vi "Set google_protobuf_Type.vi"(7 "Complete Call (T)":bool=TRUE, 8 "error in (no error)":errorcluster, 10 "package_templatemessage":T1, 11 "gRPCid":T9) -> (0 "error out":errorcluster)   [LabVIEW 2020, in "Measurement Plugin Measurement Server Internal.lvlib"]
uses:
  Measurement Plugin Measurement Server Internal.lvlib
  <vilib>/gRPC/LabVIEW gRPC Library/Shared/grpcId.ctl
  google_protobuf_Type.ctl
  google_protobuf_Field.ctl
  google_protobuf_Field_Kind.ctl
  google_protobuf_Field_Cardinality.ctl
  google_protobuf_Option.ctl
  google_protobuf_Any.ctl
  google_protobuf_SourceContext.ctl
  google_protobuf_Syntax.ctl
  google_protobuf_Type_Flat.ctl
  google_protobuf_Field_Flat.ctl
  google_protobuf_Option_Flat.ctl
  google_protobuf_Any_Flat.ctl
  google_protobuf_SourceContext_Flat.ctl
  dcc74a39-081a-4bdd-860b-8ed792803c96.vi
  RichToFlatgoogle_protobuf_Field.vi
  RichToFlatgoogle_protobuf_Option.vi
  RichToFlatgoogle_protobuf_SourceContext.vi
  <vilib>/gRPC/LabVIEW gRPC Library/Shared/TranslateGrpcError.vi
  RichToFlatgoogle_protobuf_Any.vi
  <vilib>/gRPC/LabVIEW gRPC Library/Server API/Server/Get Server DLL Path.vi
  <vilib>/Utility/error.llb/Error Cluster From Error Code.vi
  <vilib>/Utility/error.llb/Simple Error Handler.vi
  <vilib>/gRPC/LabVIEW gRPC Library/grpc-lvsupport-release.lvlib
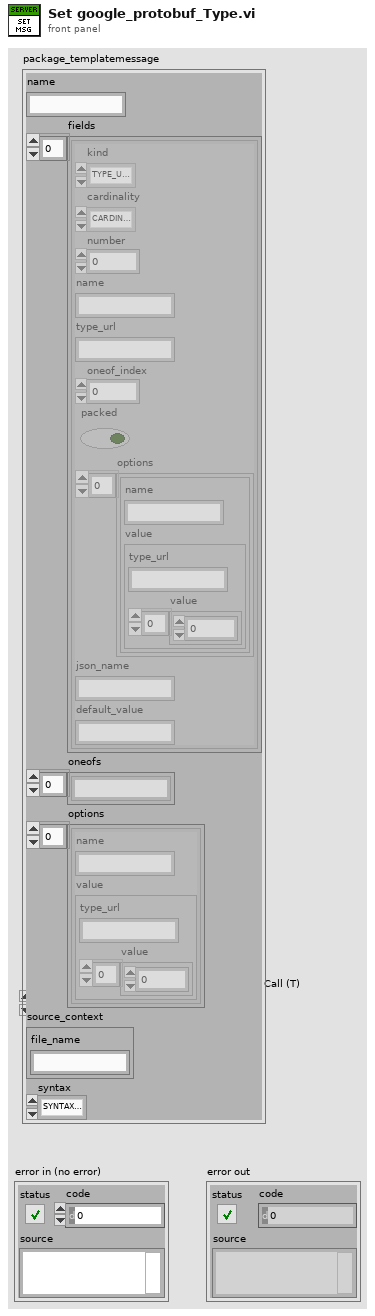
[diagram p1: front panel]
types:
  T1 = typedef "Measurement Plugin Measurement Server Internal.lvlib/google_protobuf_Type.ctl" = cluster{"name":string, "fields":T2[], "oneofs":string[], "options":T5[], "source_context":T7, "syntax":T8}
  T2 = typedef "Measurement Plugin Measurement Server Internal.lvlib/google_protobuf_Field.ctl" = cluster{"kind":T3, "cardinality":T4, "number":i32, "name":string, "type_url":string, "oneof_index":i32, "packed":bool, "options":T5[], "json_name":string, "default_value":string}
  T3 = typedef "Measurement Plugin Measurement Server Internal.lvlib/google_protobuf_Field_Kind.ctl" = enum32{"TYPE_UNKNOWN", "TYPE_DOUBLE", "TYPE_FLOAT", "TYPE_INT64", "TYPE_UINT64", "TYPE_INT32", "TYPE_FIXED64", "TYPE_FIXED32", "TYPE_BOOL", "TYPE_STRING", "TYPE_GROUP", "TYPE_MESSAGE", "TYPE_BYTES", "TYPE_UINT32", "TYPE_ENUM", "TYPE_SFIXED32", "TYPE_SFIXED64", "TYPE_SINT32", "TYPE_SINT64"}
  T4 = typedef "Measurement Plugin Measurement Server Internal.lvlib/google_protobuf_Field_Cardinality.ctl" = enum32{"CARDINALITY_UNKNOWN", "CARDINALITY_OPTIONAL", "CARDINALITY_REQUIRED", "CARDINALITY_REPEATED"}
  T5 = typedef "Measurement Plugin Measurement Server Internal.lvlib/google_protobuf_Option.ctl" = cluster{"name":string, "value":T6}
  T6 = typedef "Measurement Plugin Measurement Server Internal.lvlib/google_protobuf_Any.ctl" = cluster{"type_url":string, "value":u8[]}
  T7 = typedef "Measurement Plugin Measurement Server Internal.lvlib/google_protobuf_SourceContext.ctl" = cluster{"file_name":string}
  T8 = typedef "Measurement Plugin Measurement Server Internal.lvlib/google_protobuf_Syntax.ctl" = enum32{"SYNTAX_PROTO2", "SYNTAX_PROTO3"}
  T9 = typedef "grpc-lvsupport-release.lvlib/grpcId.ctl" = u64
  T10 = typedef "Measurement Plugin Measurement Server Internal.lvlib/google_protobuf_Type_Flat.ctl" = cluster{"name":string, "fields":T11[], "oneofs":string[], "options":T12[], "source_context":T14, "syntax":T8}
  T11 = typedef "Measurement Plugin Measurement Server Internal.lvlib/google_protobuf_Field_Flat.ctl" = cluster{"kind":T3, "cardinality":T4, "number":i32, "name":string, "type_url":string, "oneof_index":i32, "packed":bool, "options":T12[], "json_name":string, "default_value":string}
  T12 = typedef "Measurement Plugin Measurement Server Internal.lvlib/google_protobuf_Option_Flat.ctl" = cluster{"name":string, "value":T13}
  T13 = typedef "Measurement Plugin Measurement Server Internal.lvlib/google_protobuf_Any_Flat.ctl" = cluster{"type_url":string, "value":u8[]}
  T14 = typedef "Measurement Plugin Measurement Server Internal.lvlib/google_protobuf_SourceContext_Flat.ctl" = cluster{"file_name":string}
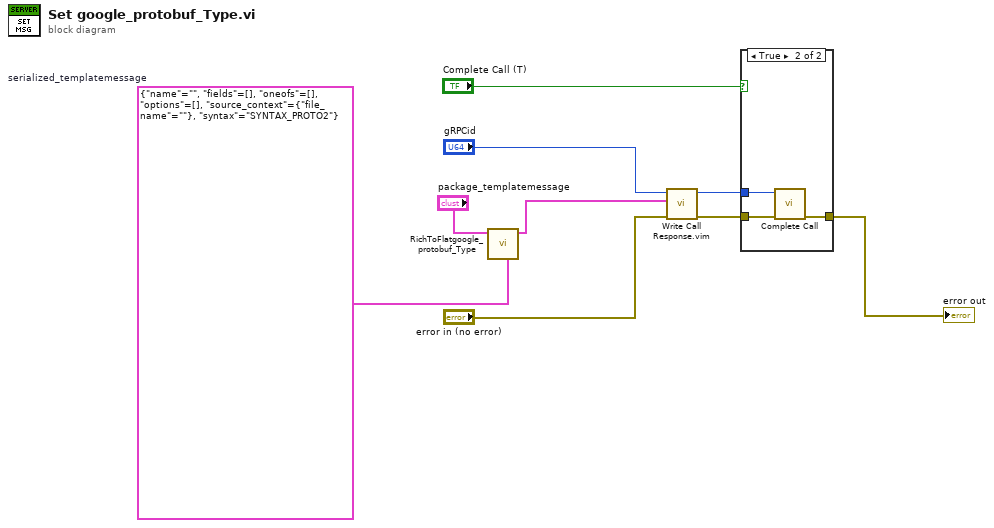
[diagram p0: block diagram]
diagram:
  w2 = T10 {"name"="", "fields"=[], "oneofs"=[], "options"=[], "source_context"={"file_name"=""}, "syntax"=enum."SYNTAX_PROTO2"}  # serialized_templatemessage
  n1 = call "RichToFlatgoogle_protobuf_Type.vi"("OutputClusterType"=w2, "InputCluster"="package_templatemessage") -> ("OutputCluster"=w1:T10)  [unwired: 9 in]
  n2 = call "Write Call Response.vim"("error in"="error in (no error)", "Response Data"=w1, "gRPCid in"="gRPCid") -> ("error out"=w6:errorcluster, "gRPCid out"=w7:T9)  [unwired: 7 in]
  n3 = case shown="True" "Complete Call (T)" {
    tunnel: [w10 w13] -> w9
    tunnel: w7 -> [_ w12]
    tunnel: w6 -> [w10 w11]
    frame False {
    }
    frame True {
      n4 = call <vilib>:"Complete Call.vi"("gRPCid"=w12, "error in"=w11) -> ("error out"=w13:errorcluster)  [unwired: 8 in]
    }
  }
  "error out" <- w9
